vi "Does config file section exist.vi"(8 "error in (no error)":errorcluster, 10 "Section name":string, 11 "file (use dialog)":path) -> (0 "error out":errorcluster, 2 "Item names":string[](array[string]), 3 "Section found?":bool)   [LabVIEW 2013]
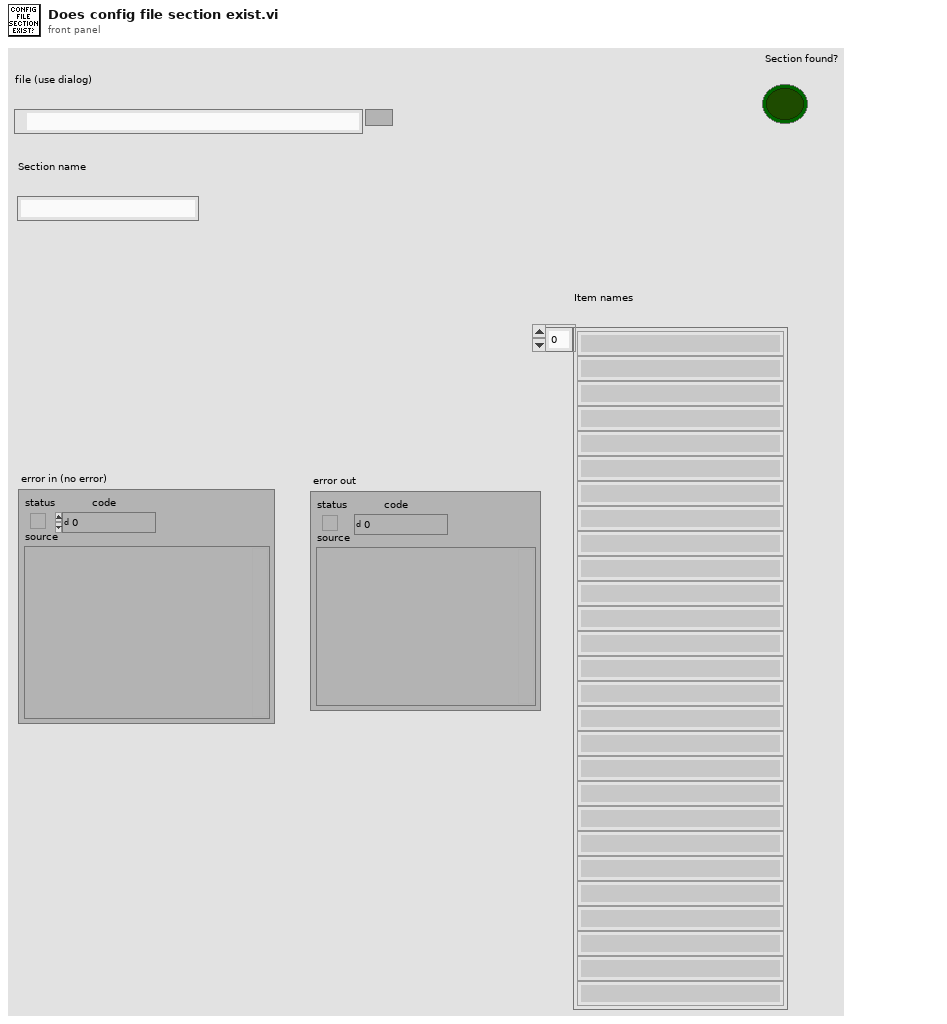
[diagram p1: front panel]
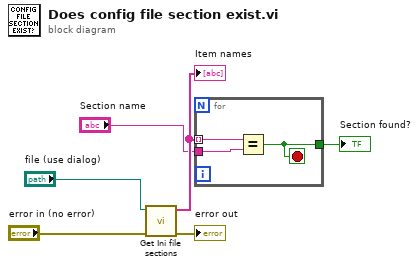
[diagram p0: block diagram]
diagram:
  n1 = call "Get Ini file sections.vi"("error in (no error)"="error in (no error)", "file (use dialog)"="file (use dialog)") -> ("error out"=→"error out":errorcluster, "Item names"=w3:string[])  [unwired: 6 in]
  "Item names" <- w3
  n2 = for {
    tunnel: w3 -> [w9] mode=indexing
    tunnel: "Section name" -> [w8]
    tunnel: [w7] -> w1
    stop <- w7 stop-if-true
    n3 = Equal?(x=w9, y=w8) -> (x = y?=w7:bool)
  }
  "Section found?" <- w1
